vi "TeleopDrive.vi"(10 "X":dbl, 11 "Y":dbl) -> ()   [LabVIEW 2015]
uses:
  Framework/Robot Global Data.vi
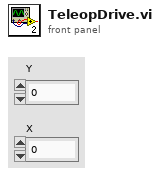
[diagram p1: front panel]
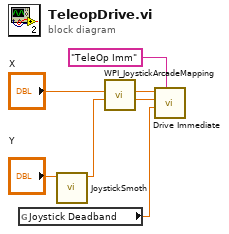
[diagram p0: block diagram]
diagram:
  n1 = global read "Robot Global Data.vi" "Joystick Deadband"() -> (w7:dbl)
  n2 = call "JoystickSmoth.vi"("joystick Value"="Y") -> ("new Joystick Value"=w1:dbl)  [unwired: 10 in]
  n3 = call <vilib>:"WPI_JoystickArcadeMapping.vi"("Y axis value"=w1, "X axis value"="X") -> ("Right Motor Value"=w6:dbl, "Left Motor Value"=w5:dbl)  [unwired: 8 in]
  n4 = call "Drive Immediate.vi"("Description"="TeleOp Imm", "Deadband Value"=w7, "Right Setpoint"=w6, "Left Setpoint"=w5) -> ()  [unwired: 7 in, 1 out]
